vi "Untitled 1.vi"() -> ()   [LabVIEW 2021, in "ELAN PDU.lvclass"]
uses:
  ELAN PDU.lvclass
  Elan channel state.ctl
panel:
  in  "ELAN PDU":T2={"target address"=0, "source address"=0, "collective state"=0, "channel state"=enum."Invalid", "command"={"type"="k", "number"=1}, "data"=[]}
  # "USED DATA\n(target address,\nsource address,\ncollective state,\nchannel state,\ncommand,\ndata)"
  # "Component address"
  # "Control system address"
  # "Command"
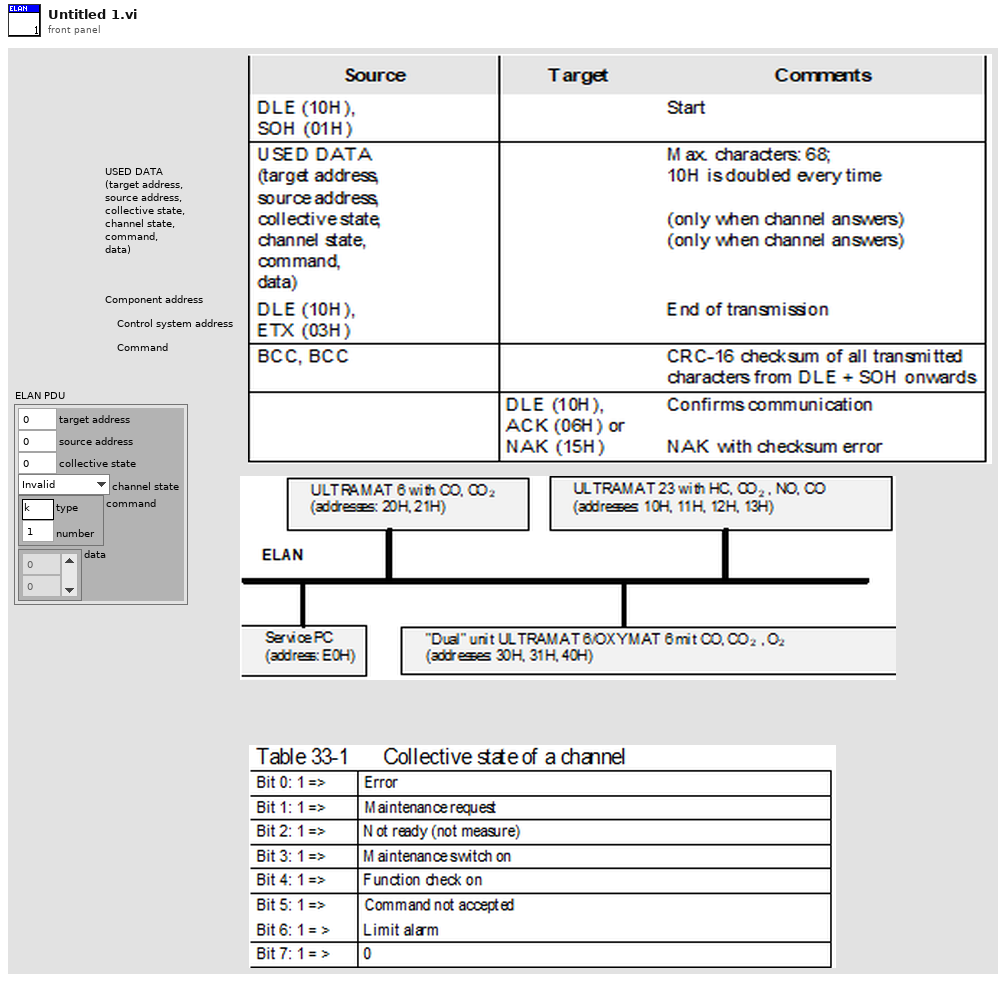
[diagram p1: front panel]
types:
  T1 = typedef "ELAN PDU.lvclass/Elan channel state.ctl" = enum16{"Invalid", "Warm-up", "Pause", "Standby", "Measure", "Zero calibration", "Adjust component slope", "Not yet defined1", "Adjust curve dip", "Adjust linearization sensitivity", "Adjust temperature compensation", "Adjust pressure compensation", "Adjust linearization zero", "Not yet defined2", "Autocal", "Adjust phase", "Zero calibration of O2 sensor", "Synchronous zero calibration", "Purging for synchronous zero calibration", "Adjust analog output", "Adjust analog input", "Autocal check"}
  T2 = cluster{"target address":u8, "source address":u8, "collective state":u8, "channel state":T1, "command":cluster{"type":string, "number":u8}, "data":u8[]}
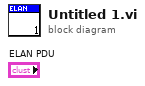
[diagram p0: block diagram]
diagram:
